vi "Edge Detection.vi"(10 "button":bool) -> (2 "risingEdge":bool)   [LabVIEW 2016]
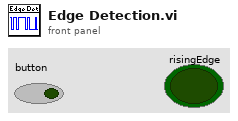
[diagram p1: front panel]
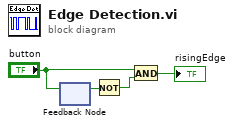
[diagram p0: block diagram]
diagram:
  n1 = feedback-in #1("button") -> ()
  n2 = feedback #1() -> (w2:bool)  [unwired: 1 in]
  n3 = Not(x=w2) -> (.not. x?=w1:bool)
  n4 = And(x="button", y=w1) -> (x .and. y?=→"risingEdge":bool)
